vi "UnzipSelectFiles-b.vi"(8 "error in (no error)":errorcluster, 9 "Target directory (same as Zip file if empty)":path, 10 "Files to Unzip":string[](array[string]), 11 "Zip file":path) -> (0 "error out":errorcluster, 2 "Preview":string, 3 "Unzipped files":path[](array[path]))   [LabVIEW 2020]
doc: "Unzips the contents of <B>Zip file</B> to the <B>Target directory</B>. Set <B>Preview only?</B> to TRUE to preview the list of files in <B>Zip file</B> before you unzip the zip file. This VI cannot unzip a zip file that is password protected."
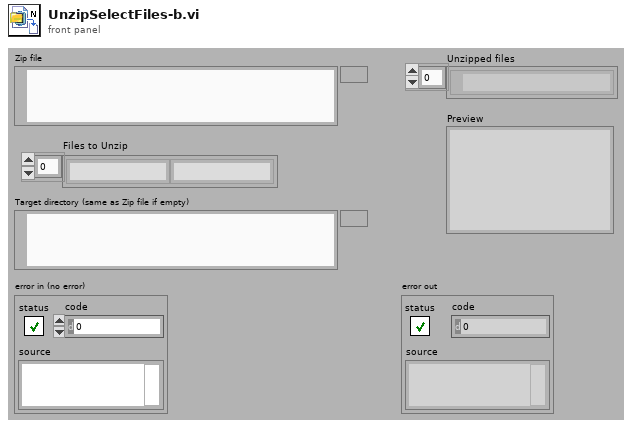
[diagram p1: front panel]
types:
  T1 = cluster{"version":u32, "version needed":u32, "flag":u32, "compression metthod":u32, "dosDate":u32, "crc":u32, "compressed size":u32, "uncompressed size":u32, "size_filename":u32, "size_file_extra":u32, "size_file_comment":u32, "disk_enum_start":u32, "internal_fa":u32, "external_fa":u32, "tmu_date":cluster{"second":u32, "minute":u32, "hour":u32, "day of month":u32, "month":u32, "year":u32}}
  T2 = enum16{"open", "replace", "create", "open or create", "replace or create", "replace or create with confirmation"}
  T3 = cluster{"second":u32, "minute":u32, "hour":u32, "day of month":u32, "month":u32, "year":u32}
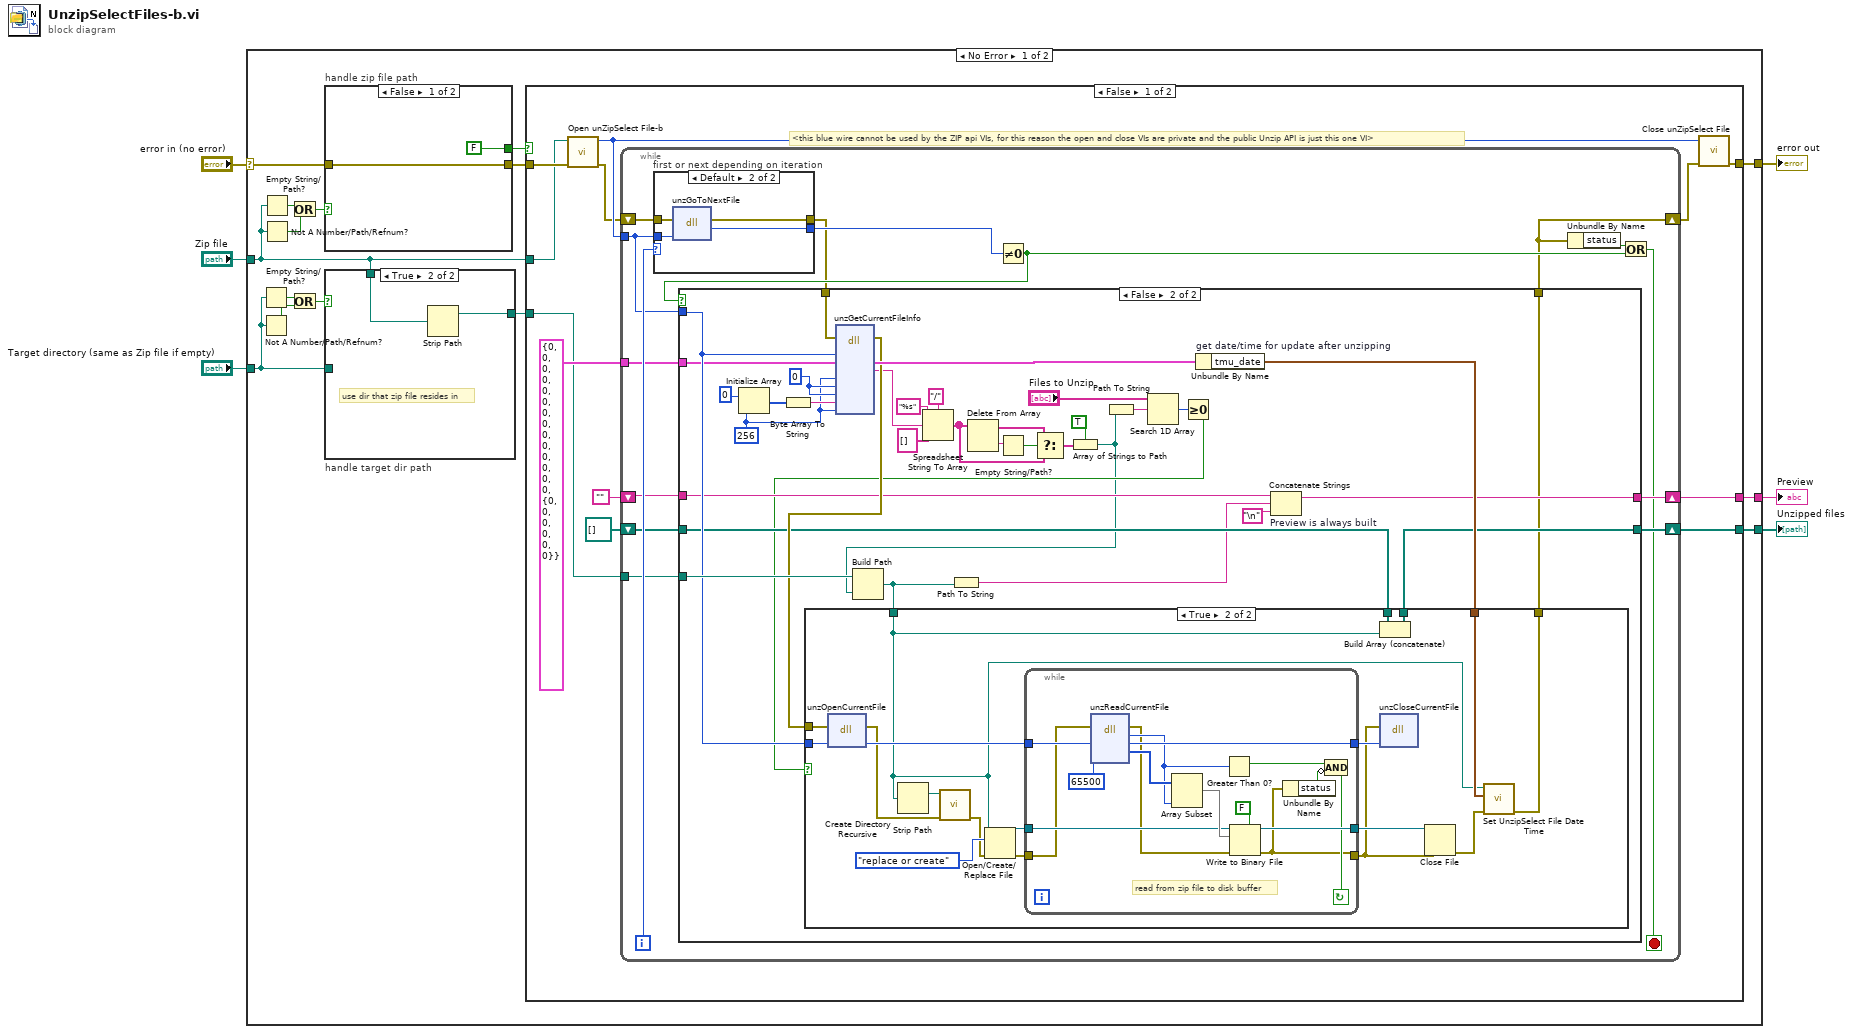
[diagram p0: block diagram]
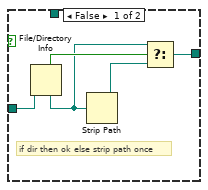
[diagram p2: hidden frame]
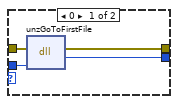
[diagram p5: hidden frame]
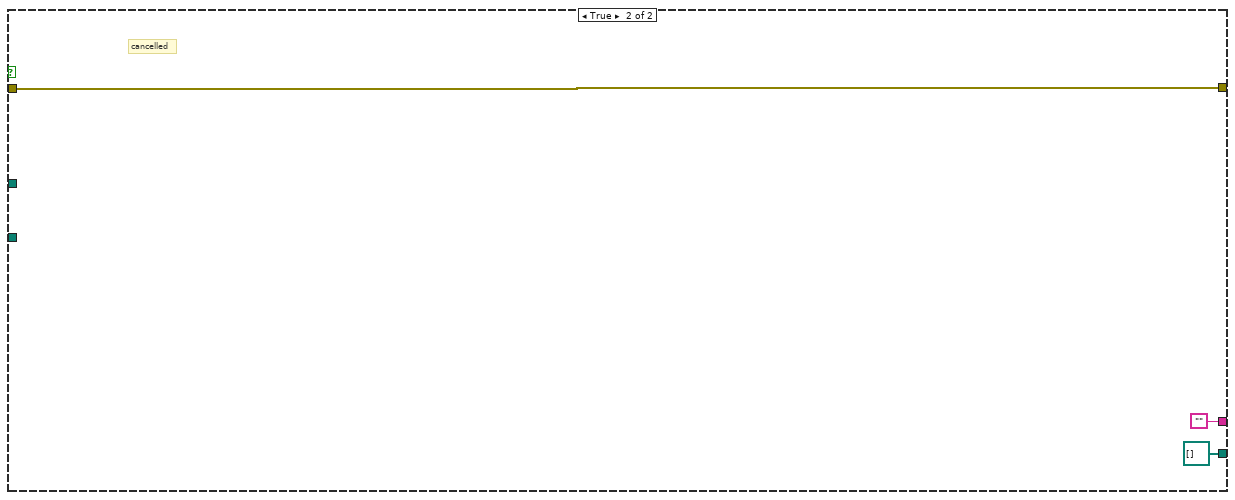
[diagram p6: hidden frame]
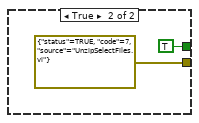
[diagram p7: hidden frame]
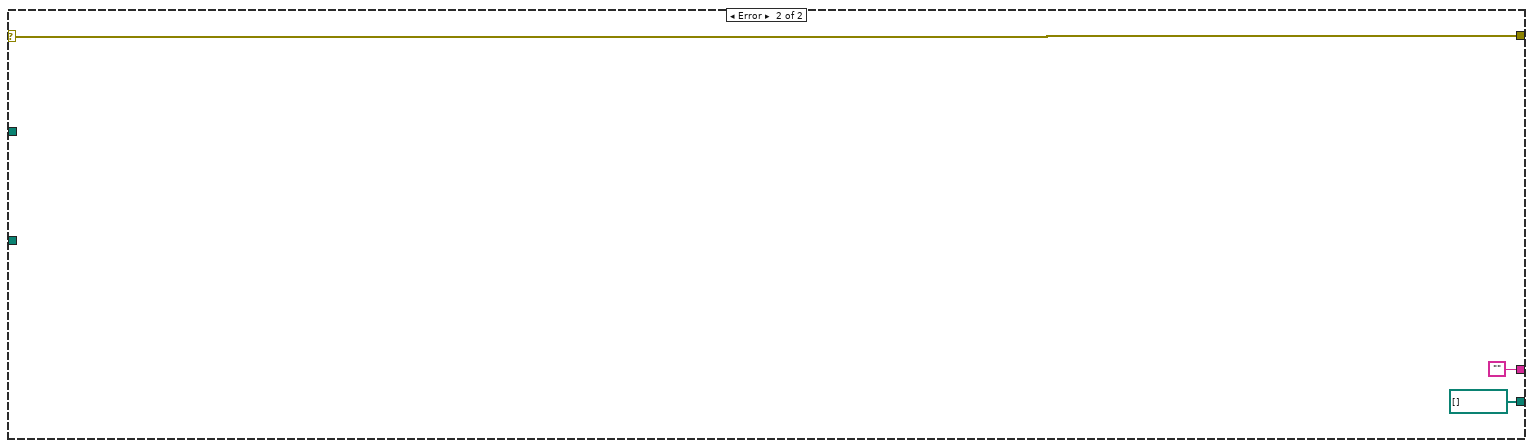
[diagram p8: hidden frame]
diagram:
  n1 = case shown="No Error" "error in (no error)" {
    selector: "error in (no error)" -> [w15 w146]
    tunnel: [w21 w146] -> w6
    tunnel: "Zip file" -> [w7 _]
    tunnel: [w19 path[] []] -> w4
    tunnel: [w16 ""] -> w3
    tunnel: "Target directory (same as Zip file if empty)" -> [w10 _]
    frame No Error {
      n2 = Empty String/Path?(string/path=w10) -> (empty?=w13:bool)
      n3 = Not A Number/Path/Refnum?(number/path/refnum=w10) -> (NaN/Path/Refnum?=w8:bool)
      n4 = Empty String/Path?(string/path=w7) -> (empty?=w20:bool)
      n5 = Not A Number/Path/Refnum?(number/path/refnum=w7) -> (NaN/Path/Refnum?=w11:bool)
      n6 = Or(x=w20, y=w11) -> (x .or. y?=w12:bool)
      n7 = Or(x=w13, y=w8) -> (x .or. y?=w9:bool)
      n8 = case "handle zip file path" shown="False" w12 {
        tunnel: [FALSE TRUE] -> w18
        tunnel: [w140 errorcluster {"status"=TRUE, "code"=7, "source"="UnzipSelectFiles.vi"} ("error constant")] -> w17
        tunnel: w15 -> [w140 _]
        frame False {
        }
        frame True {
        }
      }
      n9 = case "handle target dir path" shown="True" w9 {
        tunnel: [w25 w27] -> w14
        tunnel: w7 -> [_ w28]
        tunnel: w10 -> [w24 _]
        frame False {
          # "if dir then ok else strip path once"
          n10 = File/Directory Info(path=w24) -> (directory=w26:bool, resolved path=w23:path)  [unwired: 1 in, 5 out]
          n11 = Strip Path(path=w23) -> (stripped path=w22:path)  [unwired: 1 out]
          n12 = Select(t=w23, s=w26, f=w22) -> (s? t:f=w25:path)
        }
        frame True {
          # "use dir that zip file resides in"
          n13 = Strip Path(path=w28) -> (stripped path=w27:path)  [unwired: 1 out]
        }
      }
      n14 = case shown="False" w18 {
        tunnel: [w40 w139] -> w21
        tunnel: w7 -> [w30 _]
        tunnel: [w34 path[] []] -> w19
        tunnel: w17 -> [w33 w139]
        tunnel: [w31 ""] -> w16
        tunnel: w14 -> [w29 _]
        frame False {
          # "<this blue wire cannot be used by the ZIP api VIs, for this reason the open and close VIs are private and the public Unzip API is just this one VI>"
          n15 = call "Open unZipSelect File-b.vi"("error in (no error)"=w33, "target"=w30) -> ("error out"=w38:errorcluster, "unzip file out"=w39:i64)  [unwired: 4 in]
          n16 = while {
            tunnel: w39 -> [w52]
            shift-right: [w43] -> w37
            shift-left: w38 -> [w54]
            tunnel: T1 {"version"=0, "version needed"=0, "flag"=0, "compression metthod"=0, "dosDate"=0, "crc"=0, "compressed size"=0, "uncompressed size"=0, "size_filename"=0, "size_file_extra"=0, "size_file_comment"=0, "disk_enum_start"=0, "internal_fa"=0, "external_fa"=0, "tmu_date"={"second"=0, "minute"=0, "hour"=0, "day of month"=0, "month"=0, "year"=0}} ("pfile_info") -> [w51]
            tunnel: w29 -> [w50]
            shift-right: [w49] -> w34
            shift-left: path[] [] -> [w48]
            shift-right: [w46] -> w31
            shift-left: "" -> [w45]
            i -> [w55]
            stop <- w42 stop-if-true
            n17 = case "first or next depending on iteration" shown="Default" w55 {
              tunnel: w52 -> [w132 w134]
              tunnel: w54 -> [w131 w136]
              tunnel: [w130 w135] -> w44
              tunnel: [w129 w133] -> w53
              frame 0 {
                n18 = dll-call lib="LabVIEW" fn="unzGoToFirstFile"(error in=w131, "file"=w132) -> (error out=w130:errorcluster, "return type"=w129:i16)  [unwired: 3 in, 1 out]
              }
              frame Default {
                n19 = dll-call lib="LabVIEW" fn="unzGoToNextFile"(error in=w136, "file"=w134) -> (error out=w135:errorcluster, "return type"=w133:i16)  [unwired: 3 in, 1 out]
              }
            }
            n20 = Not Equal To 0?(x=w53) -> (x != 0?=w47:bool)
            n21 = case shown="False" w47 {
              tunnel: w52 -> [_ w91]
              tunnel: w51 -> [_ w89]
              tunnel: w50 -> [_ w92]
              tunnel: [w58 w85] -> w49
              tunnel: w48 -> [w58 w86]
              tunnel: [w57 w84] -> w46
              tunnel: w45 -> [w57 w83]
              tunnel: [w56 w75] -> w43
              tunnel: w44 -> [w56 w74]
              frame True {
                # "no more files or none to begin with"
              }
              frame False {
                w77 = u32 256 ("fileNameBufferSize")
                w93 = 0 ("pfile_info")
                n22 = Initialize Array(u8 0, w77) -> (w79:u8[])
                n23 = Byte Array To String(unsigned byte array=w79) -> (string=w78:string)
                n24 = dll-call lib="LabVIEW" fn="unzGetCurrentFileInfo"(error in=w74, "file"=w91, "pfile_info"=w89, "fileNameBufferSize"=w77, "extraField"=w93, "extraFieldBufferSize"=w93, "szComment"=w78, "commentBufferSize"=w77) -> (error out=w87:errorcluster, "pfile_info"=w90:T1, "szFileName"=w65:string)  [unwired: 6 in, 5 out]
                n25 = Spreadsheet String To Array(delimiter (Tab)="/", format string="%s", spreadsheet string=w65, array type (2D Dbl)=string[] []) -> (array=w61:string[])
                n26 = Delete From Array(array=w61) -> (deleted portion=w70:string, array with subset deleted=w69:string[])  [unwired: 2 in]
                n27 = Empty String/Path?(string/path=w70) -> (empty?=w66:bool)
                n28 = Select(t=w69, s=w66, f=w61) -> (s? t:f=w68:string[])
                n29 = Array of Strings to Path(0:w68, 1:TRUE ("relative")) -> (2:w60:path)
                n30 = Build Path(base path=w92, name or relative path=w60) -> (appended path=w82:path)
                n31 = Path To String(path=w82) -> (string=w81:string)
                n32 = Path To String(path=w60) -> (string=w59:string)
                n33 = Search 1D Array(1D array="Files to Unzip", element=w59) -> (index of element=w63:i32)  [unwired: 1 out]
                n34 = Greater Or Equal To 0?(x=w63) -> (x >= 0?=w62:bool)
                n35 = Unbundle By Name "get date/time for update after unzipping"(w90) -> ("tmu_date"=w88:T3)
                n36 = case shown="True" w62 {
                  tunnel: w91 -> [_ w113]
                  tunnel: w88 -> [_ w104]
                  tunnel: w82 -> [_ w101]
                  tunnel: w87 -> [w94 w102]
                  tunnel: w86 -> [w95 w100]
                  tunnel: [w95 w99] -> w85
                  tunnel: [w94 w96] -> w75
                  frame False {
                    # "preview only"
                  }
                  frame True {
                    n37 = dll-call lib="LabVIEW" fn="unzOpenCurrentFile"(error in=w102, "file"=w113) -> (error out=w98:errorcluster, "file"=w112:i64)  [unwired: 2 in, 2 out]
                    n38 = Strip Path(path=w101) -> (stripped path=w106:path)  [unwired: 1 out]
                    n39 = call <vilib>:"Create Directory Recursive.vi"("error in (no error)"=w98, "directory"=w106) -> ("error out"=w105:errorcluster)  [unwired: 1 in, 4 out]
                    n40 = Open/Create/Replace File(file path (use dialog)=w101, error in=w105, operation (0:open)=T2."replace or create") -> (refnum out=w109:refnum<file>, error out=w107:errorcluster)  [unwired: 4 out]
                    n41 = while {
                      tunnel: w112 -> [w128]
                      tunnel: [w126] -> w111
                      tunnel: w109 -> [w124]
                      tunnel: [w123] -> w108
                      tunnel: w107 -> [w116]
                      tunnel: [w114] -> w97
                      stop <- w119 continue-if-true
                      # "read from zip file to disk buffer"
                      n42 = dll-call lib="LabVIEW" fn="unzReadCurrentFile"(error in=w116, "file"=w128, "len"=u32 65500) -> (error out=w115:errorcluster, "return type"=w121:i32, "file"=w126:i64, "buf"=w127:u8[])  [unwired: 3 in, 2 out]
                      n43 = Array Subset(array=w127, length=w121) -> (w125:u8[])  [unwired: 1 in]
                      n44 = Greater Than 0?(x=w121) -> (x > 0?=w117:bool)
                      n45 = Write to Binary File(file (use dialog)=w124, data=w125, error in=w115, 5:FALSE ("prepend array or string size? (T)")) -> (refnum out=w123:refnum<file>, error out=w114:errorcluster)  [unwired: 3 out]
                      n46 = Unbundle By Name(w114) -> ("status"=w118:bool)
                      n47 = Compound Arithmetic op=AND(w117, invert w118) -> (w119:bool)
                    }
                    n48 = Build Array (concatenate)(w100, w101) -> (w99:path[])
                    n49 = dll-call lib="LabVIEW" fn="unzCloseCurrentFile"(error in=w97, "file"=w111) -> ()  [unwired: 3 in, 3 out]
                    n50 = Close File(refnum=w108, error in=w97) -> (error out=w103:errorcluster)  [unwired: 1 out]
                    n51 = call "Set UnzipSelect File Date Time.vi"("error in (no error)"=w103, "Date_Time"=w104, "Path"=w101) -> ("error out"=w96:errorcluster)  [unwired: 7 out]
                  }
                }
                n52 = Concatenate Strings "Preview is always built"(w83, w81, "\n") -> (w84:string)
              }
            }
            n53 = Unbundle By Name(w43) -> ("status"=w41:bool)
            n54 = Or(x=w41, y=w47) -> (x .or. y?=w42:bool)
          }
          n55 = call "Close unZipSelect File.vi"("error in (no error)"=w37, "unzip file in"=w39) -> ("error out"=w40:errorcluster)  [unwired: 5 out]
        }
        frame True {
          # "cancelled"
        }
      }
    }
    frame Error {
    }
  }
  "error out" <- w6
  "Unzipped files" <- w4
  "Preview" <- w3
